vi "Scala Letture NI.vi"(8 "soglia % filtro":dbl=1.0 format="%#_13g", 9 "Array Settings":dbl[](array[numeric]), 10 "FILTRO":bool, 11 "Cluster READ NI in":T1 {"AI (4-20mA)"."AI 15" format="%#_6f"; "AI (4-20mA)"."AI 14" format="%#_6f"; "AI (4-20mA)"."AI 13" format="%#_6f"; "AI (4-20mA)"."AI 11" format="%#_6f"; "AI (4-20mA)"."AI 10" format="%#_6f"; "AI (4-20mA)"."AI 9" format="%#_6f"; "AI (4-20mA)"."AI 4" format="%#_6f"; "AI (4-20mA)"."AI 12" format="%#_6f"; "AI (4-20mA)"."AI 0" format="%#_6f"; "AI (4-20mA)"."AI 1" format="%#_6f"; "AI (4-20mA)"."AI 2" format="%#_6f"; "AI (4-20mA)"."AI 3" format="%#_6f"; "AI (4-20mA)"."AI 5" format="%#_6f"; "AI (4-20mA)"."AI 6" format="%#_6f"; "AI (4-20mA)"."AI 7" format="%#_6f"; "AI (4-20mA)"."AI 8" format="%#_6f"; "AI (0-10V)"."AI 31" format="%#_6f"; "AI (0-10V)"."AI 30" format="%#_6f"; "AI (0-10V)"."AI 29" format="%#_6f"; "AI (0-10V)"."AI 28" format="%#_6f"; "AI (0-10V)"."AI 27" format="%#_6f"; "AI (0-10V)"."AI 26" format="%#_6f"; "AI (0-10V)"."AI 25" format="%#_6f"; "AI (0-10V)"."AI 24" format="%#_6f"; "AI (0-10V)"."AI 23" format="%#_6f"; "AI (0-10V)"."AI 22" format="%#_6f"; "AI (0-10V)"."AI 21" format="%#_6f"; "AI (0-10V)"."AI 20" format="%#_6f"; "AI (0-10V)"."AI 19" format="%#_6f"; "AI (0-10V)"."AI 18" format="%#_6f"; "AI (0-10V)"."AI 17" format="%#_6f"; "AI (0-10V)"."AI 16" format="%#_6f"; "AI (0-10V)"."AI 15" format="%#_6f"; "AI (0-10V)"."AI 14" format="%#_6f"; "AI (0-10V)"."AI 13" format="%#_6f"; "AI (0-10V)"."AI 11" format="%#_6f"; "AI (0-10V)"."AI 10" format="%#_6f"; "AI (0-10V)"."AI 9" format="%#_6f"; "AI (0-10V)"."AI 12" format="%#_6f"; "AI (0-10V)"."AI 8" format="%#_6f"}) -> (3 "Cluster READ NI out":T1 {"AI (4-20mA)"."AI 15" format="%#_6f"; "AI (4-20mA)"."AI 14" format="%#_6f"; "AI (4-20mA)"."AI 13" format="%#_6f"; "AI (4-20mA)"."AI 11" format="%#_6f"; "AI (4-20mA)"."AI 10" format="%#_6f"; "AI (4-20mA)"."AI 9" format="%#_6f"; "AI (4-20mA)"."AI 4" format="%#_6f"; "AI (4-20mA)"."AI 12" format="%#_6f"; "AI (4-20mA)"."AI 0" format="%#_6f"; "AI (4-20mA)"."AI 1" format="%#_6f"; "AI (4-20mA)"."AI 2" format="%#_6f"; "AI (4-20mA)"."AI 3" format="%#_6f"; "AI (4-20mA)"."AI 5" format="%#_6f"; "AI (4-20mA)"."AI 6" format="%#_6f"; "AI (4-20mA)"."AI 7" format="%#_6f"; "AI (4-20mA)"."AI 8" format="%#_6f"; "AI (0-10V)"."AI 31" format="%#_6f"; "AI (0-10V)"."AI 30" format="%#_6f"; "AI (0-10V)"."AI 29" format="%#_6f"; "AI (0-10V)"."AI 28" format="%#_6f"; "AI (0-10V)"."AI 27" format="%#_6f"; "AI (0-10V)"."AI 26" format="%#_6f"; "AI (0-10V)"."AI 25" format="%#_6f"; "AI (0-10V)"."AI 24" format="%#_6f"; "AI (0-10V)"."AI 23" format="%#_6f"; "AI (0-10V)"."AI 22" format="%#_6f"; "AI (0-10V)"."AI 21" format="%#_6f"; "AI (0-10V)"."AI 20" format="%#_6f"; "AI (0-10V)"."AI 19" format="%#_6f"; "AI (0-10V)"."AI 18" format="%#_6f"; "AI (0-10V)"."AI 17" format="%#_6f"; "AI (0-10V)"."AI 16" format="%#_6f"; "AI (0-10V)"."AI 15" format="%#_6f"; "AI (0-10V)"."AI 14" format="%#_6f"; "AI (0-10V)"."AI 13" format="%#_6f"; "AI (0-10V)"."AI 11" format="%#_6f"; "AI (0-10V)"."AI 10" format="%#_6f"; "AI (0-10V)"."AI 9" format="%#_6f"; "AI (0-10V)"."AI 12" format="%#_6f"; "AI (0-10V)"."AI 8" format="%#_6f"})   [LabVIEW 2019]
uses:
  Globals.vi
  TypeDef/Cluster NI.ctl
  cDAQ_PLC Folder/controls/StatoAO_cdaq.ctl
  cDAQ_PLC Folder/controls/statoDO_Cdaq.ctl
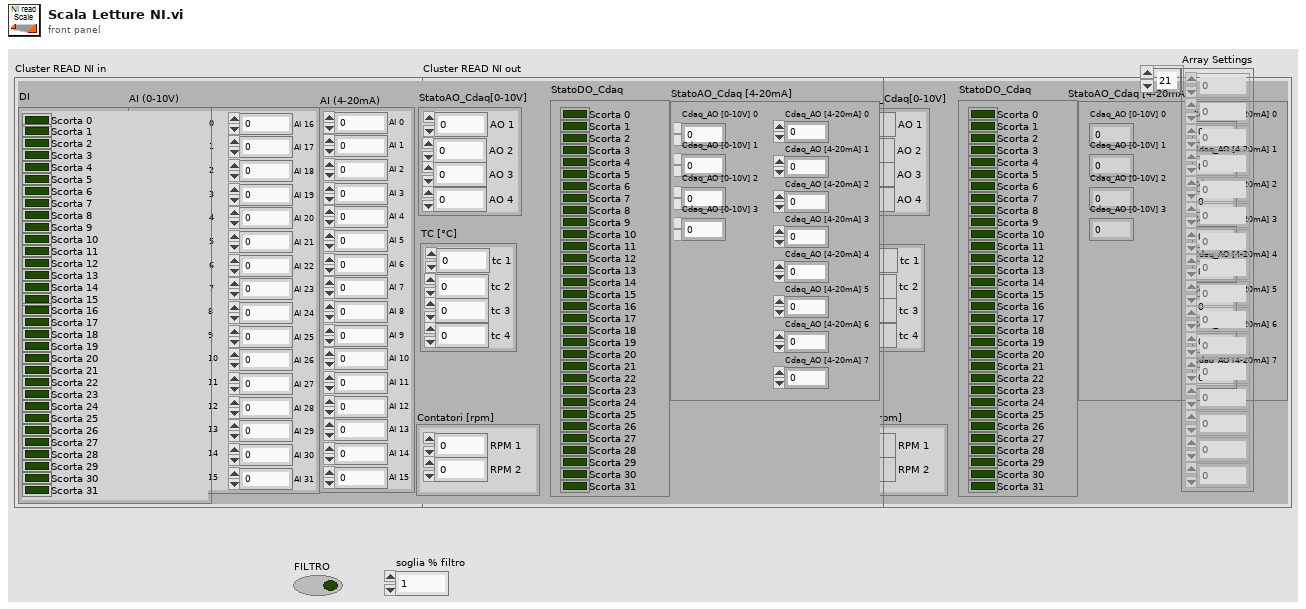
[diagram p1: front panel]
types:
  T1 = typedef "Cluster NI.ctl" = cluster{"AI (0-10V)":cluster{"AI 0":dbl, "AI 1":dbl, "AI 2":dbl, "AI 3":dbl, "AI 4":dbl, "AI 5":dbl, "AI 6":dbl, "AI 7":dbl, "AI 8":dbl, "AI 9":dbl, "AI 10":dbl, "AI 11":dbl, "AI 12":dbl, "AI 13":dbl, "AI 14":dbl, "AI 15":dbl, "AI 16":dbl, "AI 17":dbl, "AI 18":dbl, "AI 19":dbl, "AI 20":dbl, "AI 21":dbl, "AI 22":dbl, "AI 23":dbl, "AI 24":dbl, "AI 25":dbl, "AI 26":dbl, "AI 27":dbl, "AI 28":dbl, "AI 29":dbl, "AI 30":dbl, "AI 31":dbl}, "StatoAO_Cdaq[0-10V]":cluster{"AO 1":dbl, "AO 2":dbl, "AO 3":dbl, "AO 4":dbl}, "Contatori [rpm]":cluster{"RPM 1":dbl, "RPM 2":dbl}, "StatoAO_Cdaq [4-20mA]":T2, "StatoDO_Cdaq":T3, "DI":cluster{"Scorta 0":bool, "Scorta 1":bool, "Scorta 2":bool, "Scorta 3":bool, "Scorta 4":bool, "Scorta 5":bool, "Scorta 6":bool, "Scorta 7":bool, "Scorta 8":bool, "Scorta 9":bool, "Scorta 10":bool, "Scorta 11":bool, "Scorta 12":bool, "Scorta 13":bool, "Scorta 14":bool, "Scorta 15":bool, "Scorta 16":bool, "Scorta 17":bool, "Scorta 18":bool, "Scorta 19":bool, "Scorta 20":bool, "Scorta 21":bool, "Scorta 22":bool, "Scorta 23":bool, "Scorta 24":bool, "Scorta 25":bool, "Scorta 26":bool, "Scorta 27":bool, "Scorta 28":bool, "Scorta 29":bool, "Scorta 30":bool, "Scorta 31":bool}, "AI (4-20mA)":cluster{"AI 0":dbl, "AI 1":dbl, "AI 2":dbl, "AI 3":dbl, "AI 4":dbl, "AI 5":dbl, "AI 6":dbl, "AI 7":dbl, "AI 8":dbl, "AI 9":dbl, "AI 10":dbl, "AI 11":dbl, "AI 12":dbl, "AI 13":dbl, "AI 14":dbl, "AI 15":dbl}, "TC [°C]":cluster{"tc 1":dbl, "tc 2":dbl, "tc 3":dbl, "tc 4":dbl}}
  T2 = typedef "StatoAO_cdaq.ctl" = cluster{"Cdaq_AO [0-10V] 0":dbl, "Cdaq_AO [0-10V] 1":dbl, "Cdaq_AO [0-10V] 2":dbl, "Cdaq_AO [0-10V] 3":dbl, "Cdaq_AO [4-20mA] 0":dbl, "Cdaq_AO [4-20mA] 1":dbl, "Cdaq_AO [4-20mA] 2":dbl, "Cdaq_AO [4-20mA] 3":dbl, "Cdaq_AO [4-20mA] 4":dbl, "Cdaq_AO [4-20mA] 5":dbl, "Cdaq_AO [4-20mA] 6":dbl, "Cdaq_AO [4-20mA] 7":dbl}
  T3 = typedef "statoDO_Cdaq.ctl" = cluster{"Scorta 0":bool, "Scorta 1":bool, "Scorta 2":bool, "Scorta 3":bool, "Scorta 4":bool, "Scorta 5":bool, "Scorta 6":bool, "Scorta 7":bool, "Scorta 8":bool, "Scorta 9":bool, "Scorta 10":bool, "Scorta 11":bool, "Scorta 12":bool, "Scorta 13":bool, "Scorta 14":bool, "Scorta 15":bool, "Scorta 16":bool, "Scorta 17":bool, "Scorta 18":bool, "Scorta 19":bool, "Scorta 20":bool, "Scorta 21":bool, "Scorta 22":bool, "Scorta 23":bool, "Scorta 24":bool, "Scorta 25":bool, "Scorta 26":bool, "Scorta 27":bool, "Scorta 28":bool, "Scorta 29":bool, "Scorta 30":bool, "Scorta 31":bool}
  T4 = enum16{"INITIALIZE", "MEDIA", "MEDIA TUTTO", "RESET BUFFER"}
  T5 = cluster{"[0]":dbl, "[1]":dbl, "[2]":dbl, "[3]":dbl, "[4]":dbl, "[5]":dbl, "[6]":dbl, "[7]":dbl, "[8]":dbl, "[9]":dbl, "[10]":dbl, "[11]":dbl, "[12]":dbl, "[13]":dbl, "[14]":dbl, "[15]":dbl}
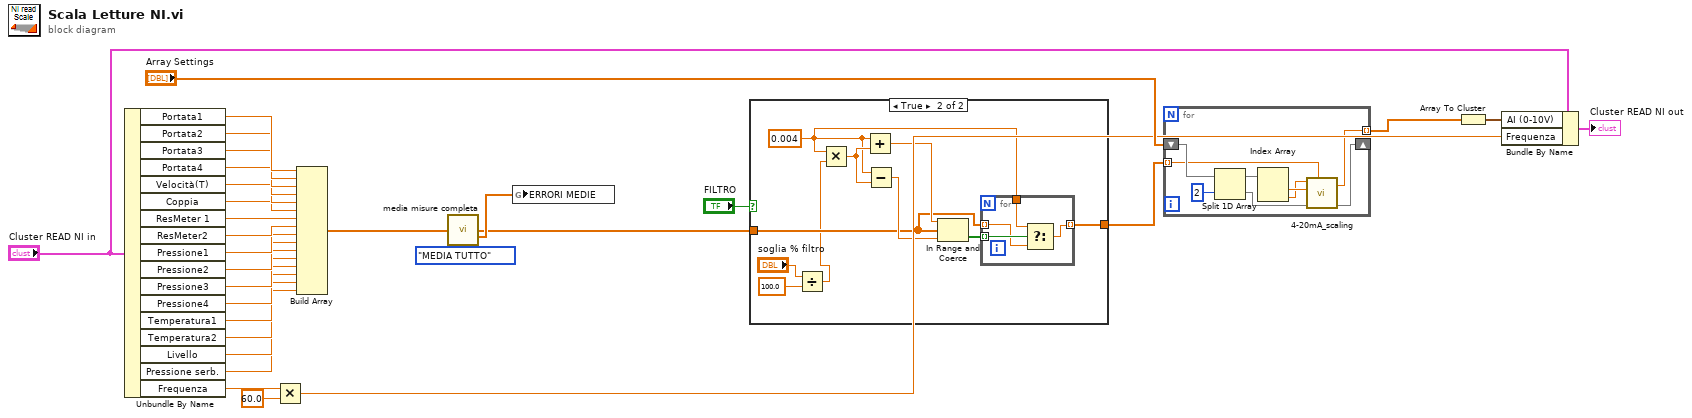
[diagram p0: block diagram]
diagram:
  n1 = Unbundle By Name("Cluster READ NI in") -> ("Portata1"=w26:dbl, "Portata2"=w25:dbl, "Portata3"=w24:dbl, "Portata4"=w23:dbl, "Velocità(T)"=w22:dbl, "Coppia"=w21:dbl, "ResMeter 1"=w20:dbl, "ResMeter2"=w19:dbl, "Pressione1"=w18:dbl, "Pressione2"=w17:dbl, "Pressione3"=w16:dbl, "Pressione4"=w15:dbl, "Temperatura1"=w14:dbl, "Temperatura2"=w13:dbl, "Livello"=w12:dbl, "Pressione serb."=w11:dbl, "Frequenza"=w10:dbl)
  n2 = Multiply(x=w10, y=60.0) -> (x*y=w7:dbl)
  n3 = Build Array(w26, w25, w24, w23, w22, w21, w20, w19, w18, w17, w16, w15, w14, w13, w12, w11) -> (w2:dbl[])
  n4 = call <userlib>:"media misure completa.vi"("Misure complete in"=w2, "Funzione"=T4."MEDIA TUTTO") -> ("Misure complete out"=w1:dbl[], "Errore%"=w3:dbl[])  [unwired: 9 in, 3 out]
  n5 = global write "Globals.vi" "ERRORI MEDIE"(w3) -> ()
  n6 = case shown="True" "FILTRO" {
    tunnel: w1 -> [w31 w35]
    tunnel: [w31 w37] -> w6
    frame False {
    }
    frame True {
      w36 = 0.004
      n7 = Divide(x="soglia % filtro", y=100.0) -> (x/y=w32:dbl)
      n8 = Multiply(x=w36, y=w32) -> (x*y=w41:dbl)
      n9 = Add(x=w36, y=w41) -> (x+y=w40:dbl)
      n10 = Subtract(x=w36, y=w41) -> (x-y=w39:dbl)
      n11 = In Range and Coerce(upper limit=w40, x=w35, lower limit=w39) -> (In Range?=w38:bool[])  [unwired: 1 out]
      n12 = for {
        tunnel: w35 -> [w42] mode=indexing
        tunnel: w38 -> [w45] mode=indexing
        tunnel: [w44] -> w37 mode=indexing
        tunnel: w36 -> [w43]
        n13 = Select(t=w43, s=w45, f=w42) -> (s? t:f=w44:dbl)
      }
    }
  }
  n14 = for {
    tunnel: w6 -> [w46] mode=indexing
    shift-right: [w51] -> _
    shift-left: "Array Settings" -> [w53]
    tunnel: [w49] -> w8 mode=indexing
    n15 = Split 1D Array(array=w53, index=2) -> (first subarray=w50:dbl[], second subarray=w51:dbl[])
    n16 = Index Array(array=w50) -> (element #1=w48:dbl, element #2=w47:dbl)  [unwired: 2 in]
    n17 = call <userlib>:"4-20mA_scaling.vi"("offset"=w47, "range"=w48, "data"=w46) -> ("scaled data"=w49:dbl)  [unwired: 3 in]
  }
  n18 = Array To Cluster(array=w8) -> (cluster=w29:T5)
  n19 = Bundle By Name(cluster="Cluster READ NI in", "AI (0-10V)"=w29, "Frequenza"=w7) -> (→"Cluster READ NI out":T1)
